vi "STM Write Meta Data (UDP Ref).vi"(4 "Address":cluster{"address":u32, "port":u16}, 6 "Options":T1={"Ignore Timeout Error"=TRUE, "timeout ms (1000)"=1000}, 7 "Meta data":T3[](array[typedef]), 8 "error in":errorcluster, 11 "connection ID":refnum<k16>) -> (0 "error out":errorcluster, 3 "Connection Info Out":T2)   [LabVIEW 2013]
doc: "Use this VI to transmit the meta data cluster to a remote computer. Sending the meta data to another computer helps maintainability since the data resides only on one side and it is shared to other computers at run time."
uses:
  stm_MetaDataElement.ctl
  stm_UDP Connection Info.ctl
  stm_UDP Write Options.ctl
  UDP/Write Meta Data (UDP Clst).vi
  NI STM.lvlib
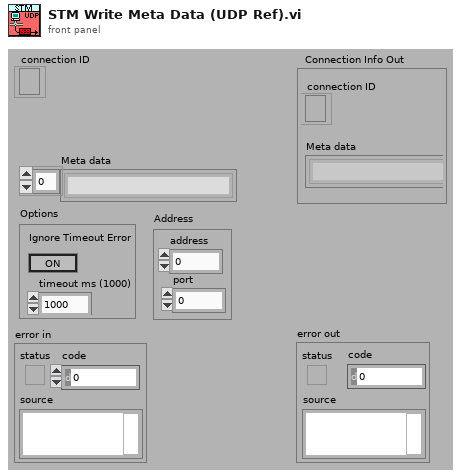
[diagram p1: front panel]
types:
  T1 = typedef "stm_UDP Write Options.ctl" = cluster{"Ignore Timeout Error":bool, "timeout ms (1000)":i32}
  T2 = typedef "stm_UDP Connection Info.ctl" = cluster{"connection ID":refnum<k16>, "Meta data":T3[]}
  T3 = typedef "stm_MetaDataElement.ctl" = string
  T4 = typedef "NI STM.lvlib/UDP Connection Info.ctl" = cluster{"connection ID":refnum<k16>, "meta data":T5[]}
  T5 = typedef "NI STM.lvlib/MetaDataElement.ctl" = string
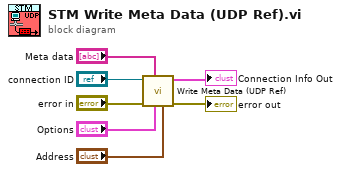
[diagram p0: block diagram]
diagram:
  n1 = call "Write Meta Data (UDP Ref).vi"("address"="Address", "options"="Options", "meta data"="Meta data", "error in"="error in", "connection ID"="connection ID") -> ("error out"=→"error out":errorcluster, "connection info out"=→"Connection Info Out":T4)  [unwired: 5 in]
